vi "zad4.vi"() -> ()   [LabVIEW 2017]
panel:
  in  "n":u64
  in  "r":dbl
  out "a(n)":dbl[](graph)
  in  "Wybierz ci¹g":enum32{"Arytmetyczny", "Geometryczny"}(radio)
  in  "a1":dbl
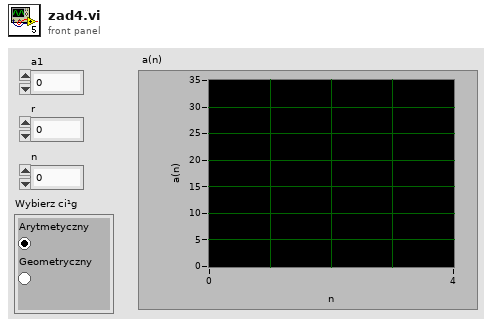
[diagram p1: front panel]
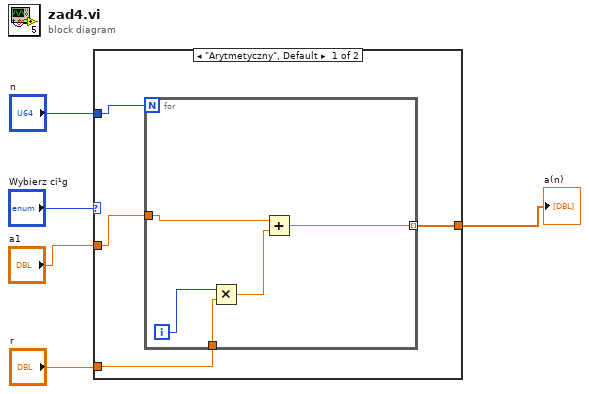
[diagram p0: block diagram]
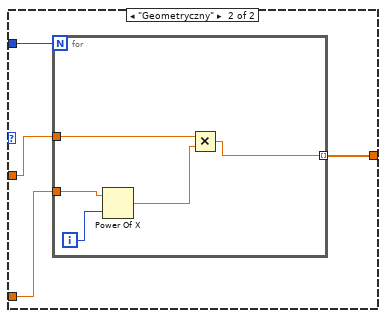
[diagram p2: hidden frame]
diagram:
  n1 = case shown="\"Arytmetyczny\", Default" "Wybierz ci¹g" {
    tunnel: "a1" -> [w9 w17]
    tunnel: "r" -> [w8 w18]
    tunnel: [w7 w16] -> w2
    tunnel: "n" -> [w6 w15]
    frame "Arytmetyczny", Default {
      n2 = for {
        N: w6 -> [_]
        tunnel: w9 -> [w14]
        tunnel: w8 -> [w11]
        tunnel: [w13] -> w7 mode=indexing
        i -> [w12]
        n3 = Multiply(x=w12, y=w11) -> (x*y=w10:dbl)
        n4 = Add(x=w14, y=w10) -> (x+y=w13:dbl)
      }
    }
    frame "Geometryczny" {
      n5 = for {
        N: w15 -> [_]
        tunnel: w18 -> [w22]
        tunnel: w17 -> [w21]
        tunnel: [w19] -> w16 mode=indexing
        i -> [w23]
        n6 = Power Of X(1:w23, 2:w22) -> (0:w20:dbl)
        n7 = Multiply(x=w21, y=w20) -> (x*y=w19:dbl)
      }
    }
  }
  "a(n)" <- w2
